vi "Instrument.Lockin.Write Configuration File.vi"(8 "error in (no error)":errorcluster, 11 "Instrument.Lockin":refnum<class "Instrument.Lockin.lvclass">) -> (0 "error out":errorcluster, 3 "Instrument.Lockin out":refnum<class "Instrument.Lockin.lvclass">)   [LabVIEW 2016, in "Instrument.Lockin.lvclass"]
uses:
  Instrument.Lockin.lvclass
  C:/Program Files (x86)/National Instruments/LabVIEW 2016/user.lib/LevyLab/Levylab Instruments/SMOs/Instrument/Instrument.lvclass
  <userlib>/LevyLab/Levylab Instruments/SMOs/Instrument/Instrument.lvclass/Instrument.ctl
  Instrument.Lockin.lvclass/Instrument.Lockin.ctl
  <userlib>/LevyLab/Levylab Instruments/SMOs/Configuration/Configuration.lvclass
  <userlib>/LevyLab/Levylab Instruments/SMOs/Instrument/Instrument.lvclass
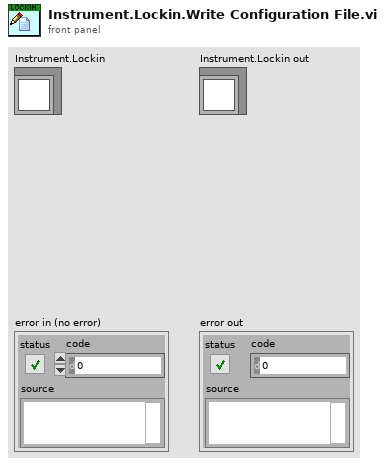
[diagram p1: front panel]
types:
  T1 = typedef "Instrument.Lockin.lvclass/Instrument.Lockin.Configuration--Cluster.ctl" = cluster{"Channels: AO":T2, "Channels: Lockin":T9, "REF Filter":cluster{"LP cutoff (Hz)":dbl, "LP prefilter":bool, "60 Hz prefilter":bool, "order":i32, "TC (s)":dbl}, "AI Configuration":cluster{"AI Configuration":T12}, "AO Configuration":cluster{"AO Configuration":T16}, "Amplifers":cluster{"offsets":dbl[], "Gain":dbl[], "Amplifiers":T19}, "DAQ":cluster{"DAQ Type":T20, "sampling":T21}, "Calibration":cluster{"Cal Info":T22[]}}
  T2 = typedef "Instrument.Lockin.lvclass/AO-cluster.ctl" = cluster{"AO Amp (V)":T3, "AO DC (V)":T4, "AO f (Hz)":T5, "AO Phase (°)":T6, "Function":T7, "I+":bool[], "Sweeping":bool[]}
  T3 = typedef "Instrument.Lockin.lvclass/AO_Amp-array.ctl" = dbl[]
  T4 = typedef "Instrument.Lockin.lvclass/AO_DC-array.ctl" = dbl[]
  T5 = typedef "Instrument.Lockin.lvclass/AO_f-array.ctl" = dbl[]
  T6 = typedef "Instrument.Lockin.lvclass/AO_phi-array.ctl" = dbl[]
  T7 = typedef "Instrument.Lockin.lvclass/Function-array.ctl" = T8[]
  T8 = typedef "Instrument.Lockin.lvclass/Function-enum.ctl" = enum16{"Sine", "Triangle", "Square", "Sawtooth"}
  T9 = typedef "Instrument.Lockin.lvclass/REF-cluster.ctl" = cluster{"REF f (Hz)":T10, "REF phi (°)":T11}
  T10 = typedef "Instrument.Lockin.lvclass/REF_f-array.ctl" = dbl[]
  T11 = typedef "Instrument.Lockin.lvclass/REF_phi-array.ctl" = dbl[]
  T12 = typedef "Instrument.Lockin.lvclass/AI.config-array.ctl" = T13[]
  T13 = typedef "Instrument.Lockin.lvclass/AI.config-cluster.ctl" = cluster{"AI.Coupling":T14, "AI.channels":tag, "AI.Range":T15}
  T14 = typedef "Instrument.Lockin.lvclass/AI.coupling-enum.ctl" = enum16{"AC", "DC", "GND"}
  T15 = typedef "Instrument.Lockin.lvclass/446xAI-enum.ctl" = enum16{"±0.316 V", "±1.00 V", "±3.16 V", "±10.0 V", "±31.6 V", "±42.4 V"}
  T16 = typedef "Instrument.Lockin.lvclass/AO.config-array.ctl" = T17[]
  T17 = typedef "Instrument.Lockin.lvclass/AO.config-cluster.ctl" = cluster{"AO.Range":T18, "AO.channels":tag}
  T18 = typedef "Instrument.Lockin.lvclass/446xAO-enum.ctl" = enum16{"±0.1 V", "±1.0 V", "±10.0 V"}
  T19 = typedef "Instrument.Lockin.lvclass/AmplifierType-enum.ctl" = enum16{"Manual", "Krohn Hite", "Femto"}
  T20 = typedef "Instrument.Lockin.lvclass/DAQType-enum.ctl" = enum16{"None", "USB 4431", "PXI 446x"}
  T21 = typedef "Instrument.Lockin.lvclass/Sampling.ctl" = cluster{"Fs":i32, "#s":i32}
  T22 = typedef "Instrument.Lockin.lvclass/Cal Info - Cluster.ctl" = cluster{"Active Device":tag, "SelfCal.LastDate/Time":timestamp, "SelfCal.LastTemp":dbl, "DevTemp":dbl, "calibration due?":bool}
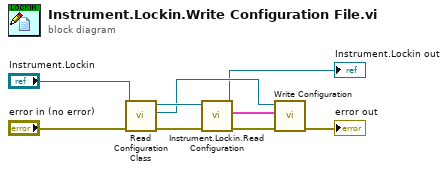
[diagram p0: block diagram]
diagram:
  n1 = call <userlib>:"Read Configuration Class.vi"("error in (no error)"="error in (no error)", "Instrument in"="Instrument.Lockin") -> ("error out"=w5:errorcluster, "Configuration.lvclass"=w8:refnum<class "Configuration.lvclass">, "Instrument out"=w9:refnum<class "Instrument.Lockin.lvclass">)  [unwired: 7 in]
  n2 = call "Instrument.Lockin.Read Configuration.vi"("error in (no error)"=w5, "Instrument.Lockin"=w9) -> ("error out"=w4:errorcluster, "Configuration"=w1:T1, "Instrument.Lockin out"=→"Instrument.Lockin out":refnum<class "Instrument.Lockin.lvclass">)  [unwired: 7 in]
  n3 = call <userlib>:"Write Configuration.vi"("error in (no error)"=w4, "Variant"=w1, "Configuration in"=w8) -> ("error out"=→"error out":errorcluster)  [unwired: 7 in, 1 out]
